vi "NPSV RTFIFO test.vi"() -> ()   [LabVIEW 2019]
uses:
  DataDef.ctl
  <vilib>/NI/Modbus Library/API/Modbus API.lvclass
  <vilib>/WPC Systems Ltd/GECO Driver/Lib/GECOBase/GECO_Driver Class/GECO_Driver.lvclass
  <vilib>/WPC Systems Ltd/GECO Driver/Lib/GECOMotion/GECOMotion/_typedefine/Axis Select.ctl
  <vilib>/WPC Systems Ltd/GECO Driver/Lib/GECOBase/GECO_Driver Class/Motion/_typedefine/GECO_Stepper Output Configuration.ctl
  <vilib>/WPC Systems Ltd/GECO Driver/Lib/GECOBase/GECO_Driver Class/Motion/_typedefine/GECO_Motion Operation Mode.ctl
  <vilib>/WPC Systems Ltd/GECO Driver/Lib/GECOBase/GECO_Driver Class/GECO_SlotName.ctl
  <vilib>/WPC Systems Ltd/GECO Driver/Lib/GECOBase/GECO_Driver Class/Motion/_typedefine/GECO_ActiveHighLow.ctl
  <vilib>/WPC Systems Ltd/GECO Driver/Lib/GECOMotion/GECOMotion/GECO Motion.lvclass
  GyroDef.ctl
  <vilib>/Platform/TimedLoop/XDataNode/timing_clust.ctl
  <vilib>/Platform/TimedLoop/XDataNode/nitl_modes.ctl
  <vilib>/Platform/TimedLoop/XDataNode/wakeup.ctl
  <vilib>/NI/Modbus Library/API/Slave/Modbus Slave.lvclass
  C:/Program Files (x86)/National Instruments/LabVIEW 2019/vi.lib/NI/Modbus Library/API/Modbus API.lvclass
  <vilib>/addons/control/pid/pid.llb/PID (DBL).vi
  <vilib>/NI/Modbus Library/API/Wrapper/Create TCP Slave.vi
  <vilib>/WPC Systems Ltd/GECO Driver/GECODriver/GECO_Initialize_RT/Initialize VIs/Initialize_GECOUnoRT_4HX.vi
  <vilib>/platform/TimedLoop/XDataNode/XDataNode.xnode
  <vilib>/addons/control/pid/NI_PID_pid.lvlib
  <vilib>/NI/Modbus Library/API/Wrapper/API Main.lvlib
  <vilib>/Platform/TimedLoop/XDataNode/XDNodeRunTimeDep.lvlib
panel:
  out "error out":errorcluster
  out "Axis 1":T1
  out "Axis 2":T1
  out "Axis 3":T1
  out "Program Period":u32
  in  "Main Setting Tab":T2(tab)
  in  "PID gains setting Tab":enum32{"Axis 1", "Axis 2", "Axis 3"}(tab)
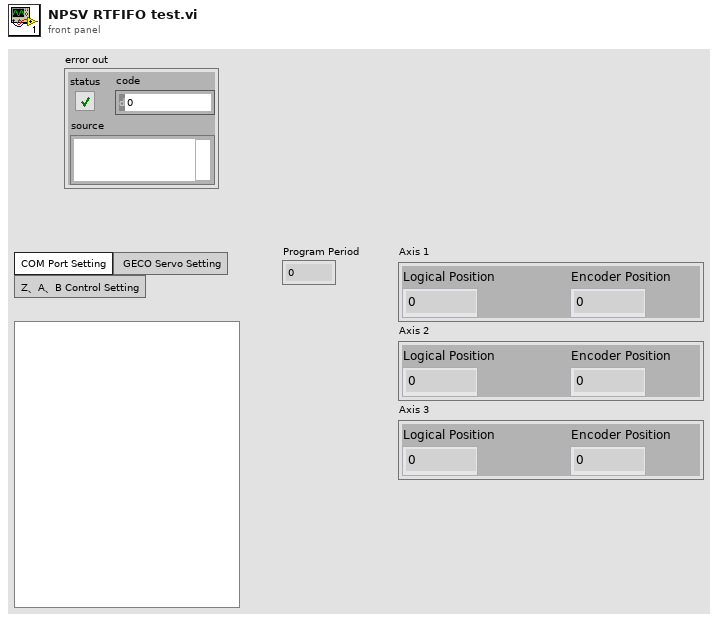
[diagram p1: front panel]
types:
  T1 = cluster{"Encoder Position":i32, "Logical Position":i32}
  T2 = enum32{"COM Port Setting", " GECO Servo Setting", "Z、A、B Control Setting"}
  T3 = typedef "DataDef.ctl" = cluster{"address starting":u16, "狀態":enum16{"初始化", "讀取", "寫入", "停止"}, "理想角度":cluster{"A":dbl, "B":dbl}, "register values":i16[], "Modbus COM":refnum<class "Modbus API.lvclass">, "TCP slave port":u16, " baud rate":u32, "Byte bits":u16, "ServoButtonControl":cluster{"三軸同退":bool, "三軸同進":bool, "三軸後退":bool, "三軸前進":bool, "二軸後退":bool, "二軸前進":bool, "一軸後退":bool, "一軸前進":bool}, "Serial Number":string, "GECO_Driver out":refnum<class "GECO_Driver.lvclass">, "number of inputs":u16, "ServoSetting":cluster{"Axis Select":T4, "Stepper Output Configuration":T5, "Motion Operation Mode":T6, "Motion Controller Slot":T7, "Singel Axis Move Paramters":cluster{"Motion Operation Mode":T6, "Target Position (0)":i32, "Velocity (10000)":i32, "Acceleration (100000)":u32, "Deacceleration (100000)":u32}, "Reverse":cluster{"Reverse Enable":bool, "Reverse Polarity":T8}, "Forward":cluster{"Forward Enable":bool, "Forward Polarity":T8}}, "GECO Motion out":refnum<class "GECO Motion.lvclass">, "Servo on":bool, "Axis 1 Position":cluster{"Encoder Position":i32, "Logical Position":i32}, "Axis 2 Position":cluster{"Encoder Position":i32, "Logical Position":i32}, "Axis 3 Position":cluster{"Encoder Position":i32, "Logical Position":i32}, "PIDSetting":cluster{"Z":i32, "A":i32, "B":i32, "Move Setting":T9, "Axis Pulse":dbl, "Axis Length":dbl, "PID gains ":cluster{"proportional gain (Kc)":dbl, "integral time (Ti, min)":dbl, "derivative time (Td, min)":dbl}}, "resource name":tag, "Save Path":refnum<file>}
  T4 = typedef "GECO Motion.lvclass/Axis Select.ctl" = enum16{"Axis 1", "Axis 2", "Axis 3", "Axis 4"}
  T5 = typedef "GECO_Driver.lvclass/GECO_Stepper Output Configuration.ctl" = enum16{"Step/Dir(One Pulse)", "CW/CCW(Two Pulse)"}
  T6 = typedef "GECO_Driver.lvclass/GECO_Motion Operation Mode.ctl" = enum16{"Absolute Position", "Relative Position", "Velocity"}
  T7 = typedef "GECO_Driver.lvclass/GECO_SlotName.ctl" = enum16{"C1", "C2", "C3", "C4"}
  T8 = typedef "GECO_Driver.lvclass/GECO_ActiveHighLow.ctl" = enum16{"Active High", "Active Low"}
  T9 = typedef "­y¸ñ.ctl" = u16
  T10 = typedef "GyroDef.ctl" = cluster{"Byte bits":u16, "baud rate":u32, "實際角度":cluster{"A":dbl, "B":dbl}, "COM Port":refnum<visa-resource-name>, "Save Path":refnum<file>}
  T11 = typedef "XDNodeRunTimeDep.lvlib/timing_clust.ctl" = cluster{"Expected End [f-1]":u64, "Actual End [f-1]":u64, "Finished Late? [f-1]":bool, "Expected End [i-1]":u64, "Actual End [i-1]":u64, "Finished Late? [i-1]":bool, "Expected Start [i]":u64, "Actual Start [i]":u64, "Expected Start [f]":u64, "Actual Start [f]":u64, "Source Name":string, "Structure Name":string, "Period":i64, "Deadline":i64, "Offset":i64, "Start":i64, "Priority":i32, "Timeout":i32, "Mode":T12, "Wakeup Reason":T13, "Error":errorcluster, "Source Type":string, "Secondary Source Type":string, "Global End Time":u64, "Global Start Time":u64, "Frame Duration":u64, "Iteration Duration":u64, "Assigned CPU":i32, "I/O Scan Engine Mode":u32}
  T12 = typedef "XDNodeRunTimeDep.lvlib/nitl_modes.ctl" = enum32{"No Change", "Process missed periods, maintain original phase", "Discard missed periods, maintain original phase", "Process missed periods, ignore original phase", "Discard missed periods, ignore original phase"}
  T13 = typedef "XDNodeRunTimeDep.lvlib/wakeup.ctl" = enum32{"Normal", "Aborted", "Asynchronous wakeup", "Timing source error", "Timed loop error", "Timeout"}
  T14 = cluster{"Motion Operation Mode":T6, "Target Position (0)":i32, "Velocity (10000)":i32, "Acceleration (100000)":u32, "Deacceleration (100000)":u32}
  T15 = cluster{"Forward Enable":bool, "Forward Polarity":T8}
  T16 = cluster{"Reverse Enable":bool, "Reverse Polarity":T8}
  T17 = cluster{"三軸同退":bool, "三軸同進":bool, "三軸後退":bool, "三軸前進":bool, "二軸後退":bool, "二軸前進":bool, "一軸後退":bool, "一軸前進":bool, "Reset Encoder Position":bool, "AlarmReset":bool}[]
  T18 = cluster{"三軸同退":bool, "三軸同進":bool, "三軸後退":bool, "三軸前進":bool, "二軸後退":bool, "二軸前進":bool, "一軸後退":bool, "一軸前進":bool, "Reset Encoder Position":bool, "AlarmReset":bool}
  T19 = enum16{"open", "replace", "create", "open or create", "replace or create", "replace or create with confirmation"}
  T20 = cluster{"Logical Position":i32, "Encoder Position":i32}
  T21 = enum16{"Step/Dir(One Pulse)", "CW/CCW(Two Pulse)"}
  T22 = enum16{"Absolute Position", "Relative Position", "Velocity"}
  T23 = cluster{"proportional gain (Kc)":dbl, "integral time (Ti, min)":dbl, "derivative time (Td, min)":dbl}
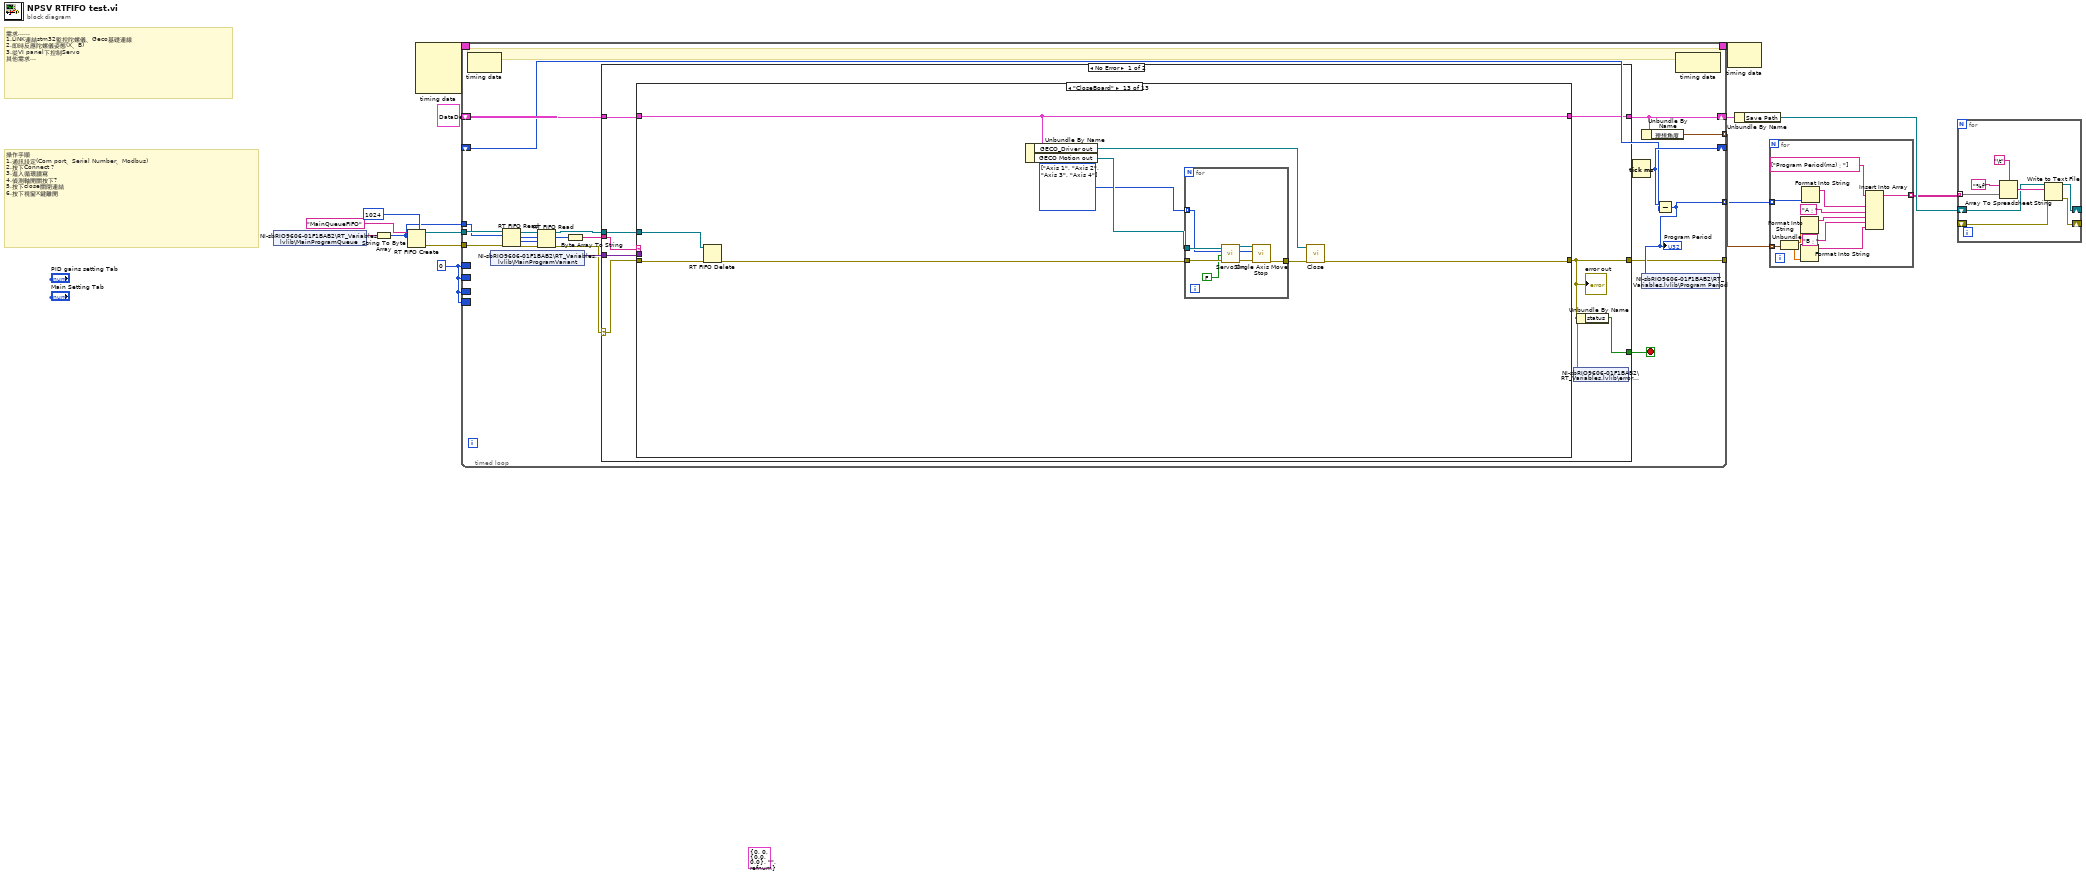
[diagram p0: block diagram]
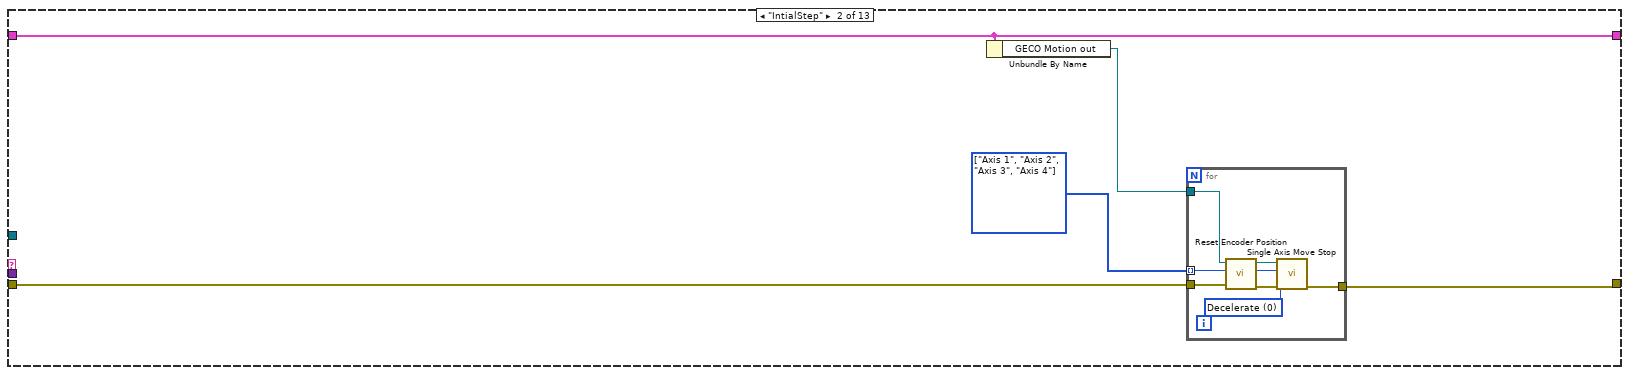
[diagram p3: hidden frame]
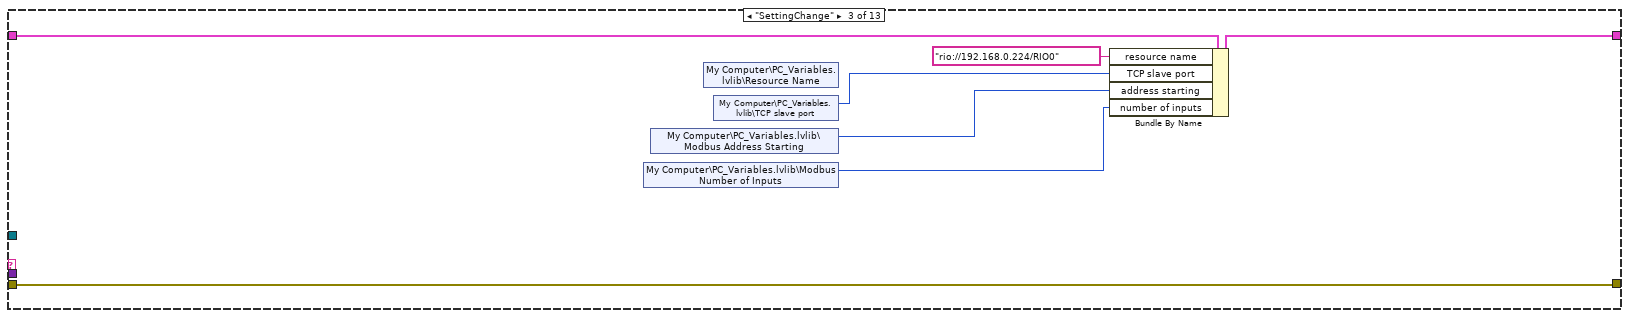
[diagram p4: hidden frame]
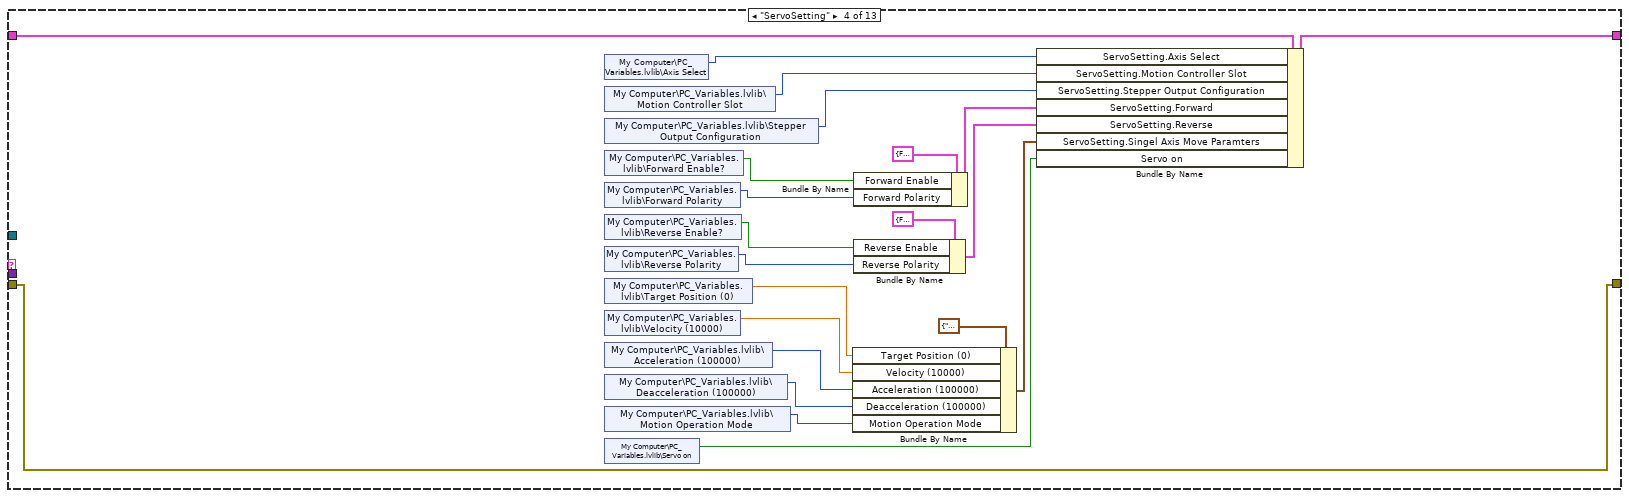
[diagram p5: hidden frame]
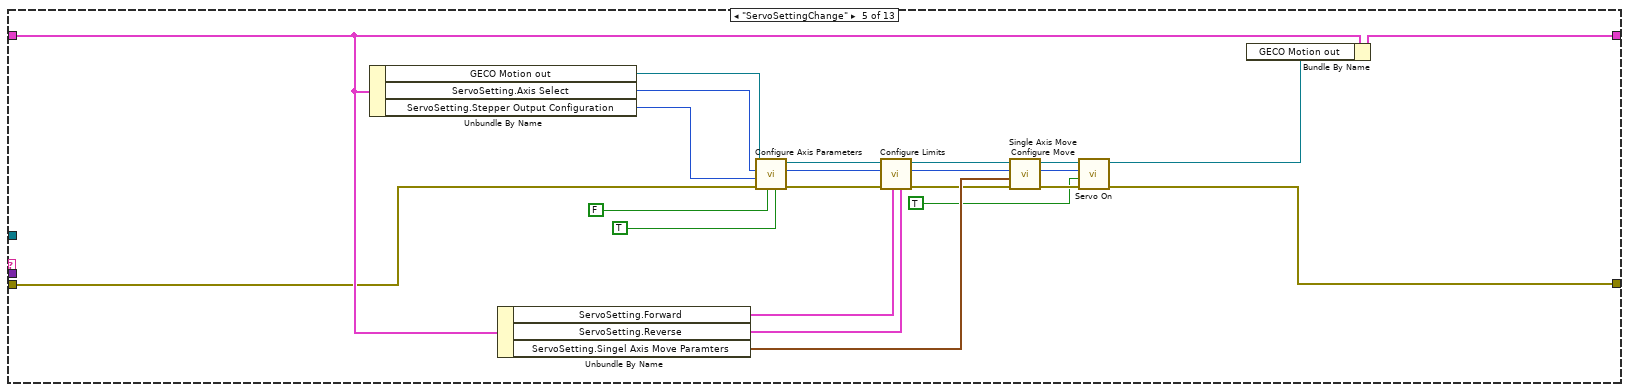
[diagram p6: hidden frame]
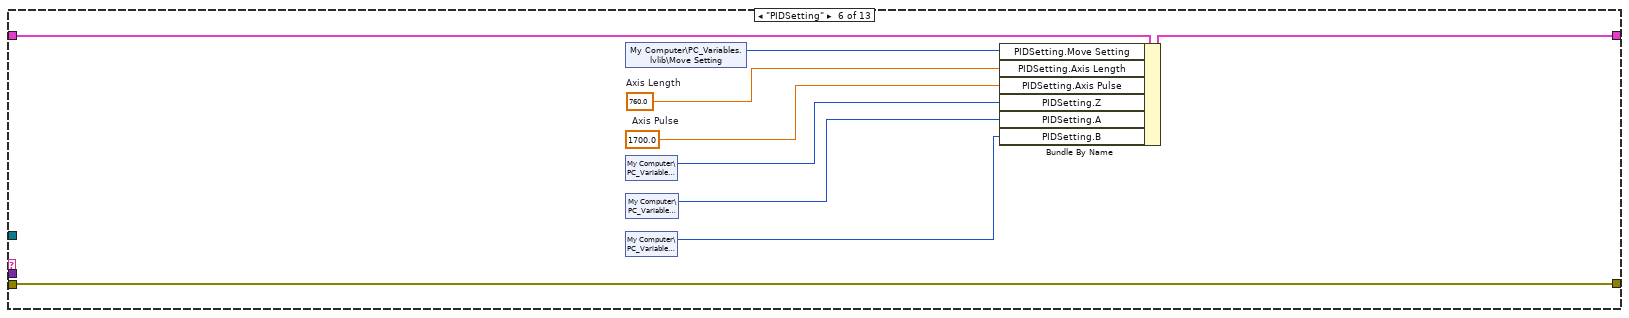
[diagram p7: hidden frame]
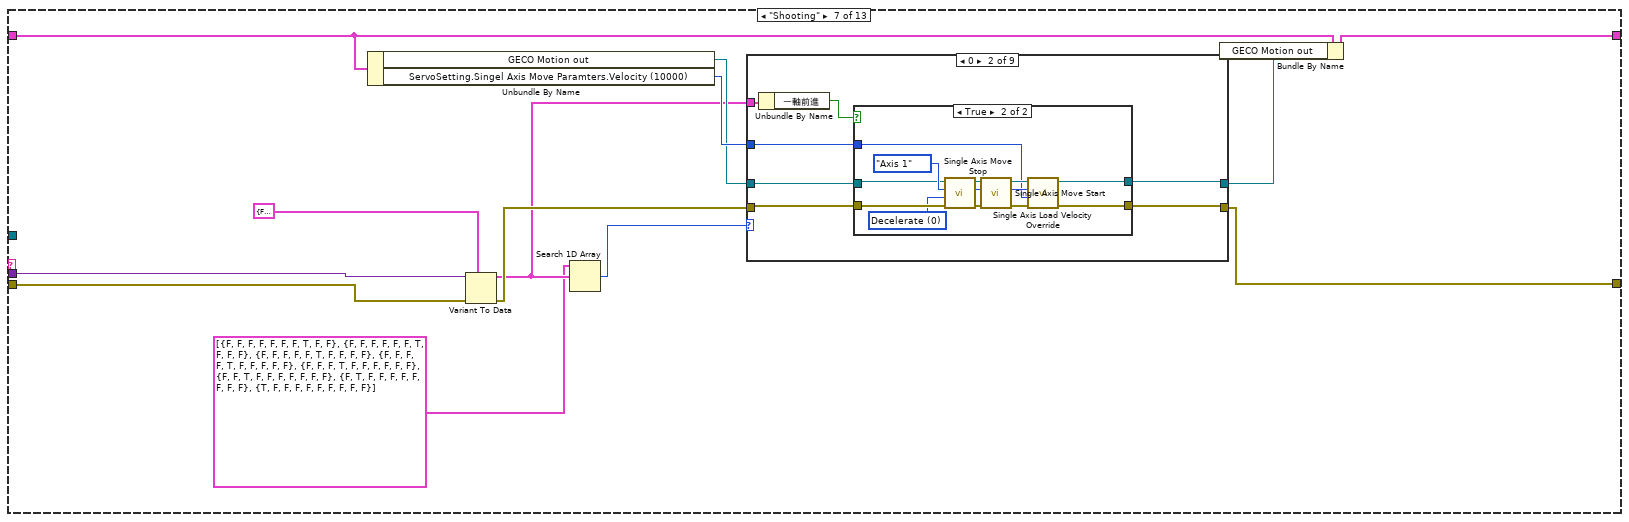
[diagram p8: hidden frame]
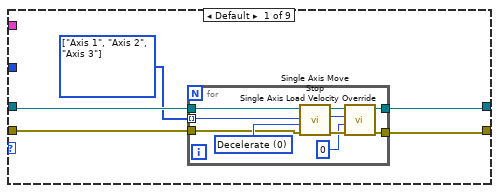
[diagram p9: hidden frame]
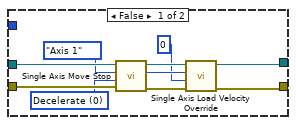
[diagram p10: hidden frame]
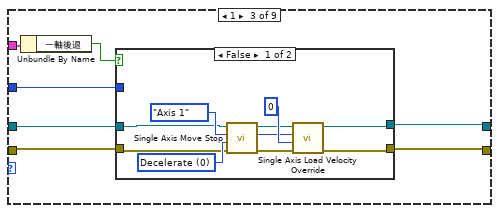
[diagram p11: hidden frame]
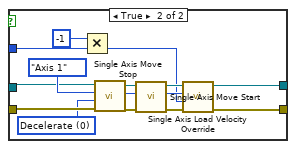
[diagram p12: hidden frame]
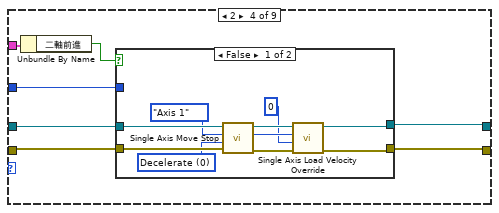
[diagram p13: hidden frame]
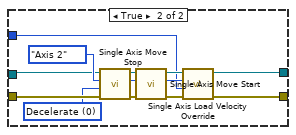
[diagram p14: hidden frame]
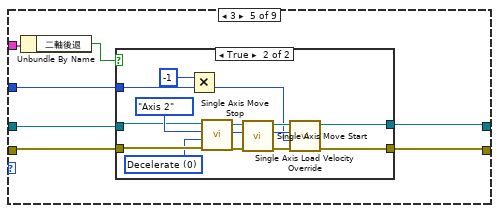
[diagram p15: hidden frame]
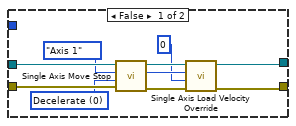
[diagram p16: hidden frame]
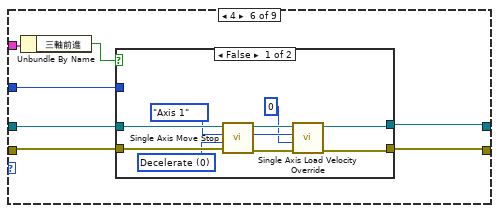
[diagram p17: hidden frame]
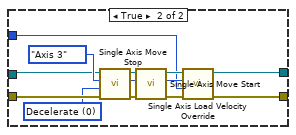
[diagram p18: hidden frame]
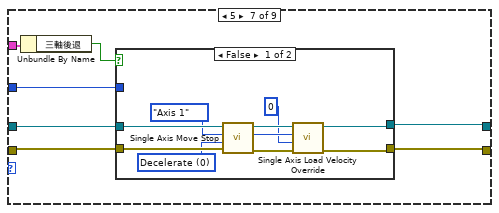
[diagram p19: hidden frame]
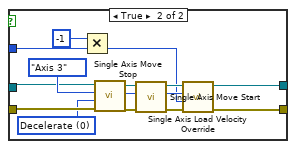
[diagram p20: hidden frame]
diagram:
  w14 = 0
  (unwired) T10 {"Byte bits"=0, "baud rate"=0, "實際角度"={"A"=0.0, "B"=0.0}, "COM Port"="", "Save Path"=refnum}
  # "操作手順\n1.通訊設定(Com port、Serial Number、Modbus)\n2.按下Connect ?\n3.進入循環讀寫\n4.偵測軸開關按下?\n5.按下close關閉連結\n6.按下視窗X鍵離開"
  # "需求......\n1.LINK連結stm32監控陀螺儀、Geco基礎連線\n2.即時反應陀螺儀姿態(X、B)\n3.從VI panel下控制Servo\n其他需求..."
  n1 = shared-variable "NI-sbRIO9606-01F1BAB2\\RT_Variables.lvlib\\MainProgramQueue"() -> (w3:string)  [unwired: 1 in, 1 out]
  n2 = String To Byte Array(string=w3) -> (unsigned byte array=w1:u8[])
  n3 = RT FIFO Create(0:"MainQueueFIFO" ("name (unnamed)"), 1:w1, 6:u32 1024 ("elements in array (1)")) -> (8:w6:refnum<k33>, 11:w2:errorcluster)  [unwired: 5 in, 1 out]
  n4 = node-c288() -> (w8:T11)  [unwired: 4 in]
  n5 = timed-loop {
    shift-right: [w31] -> w11
    shift-left: T3 {"address starting"=0, "狀態"=enum."初始化", "理想角度"={"A"=0.0, "B"=0.0}, "register values"=[], "Modbus COM"=refnum, "TCP slave port"=1, " baud rate"=0, "Byte bits"=0, "ServoButtonControl"={"三軸同退"=FALSE, "三軸同進"=FALSE, "三軸後退"=FALSE, "三軸前進"=FALSE, "二軸後退"=FALSE, "二軸前進"=FALSE, "一軸後退"=FALSE, "一軸前進"=FALSE}, "Serial Number"="", "GECO_Driver out"=refnum, "number of inputs"=0, "ServoSetting"={"Axis Select"=enum."Axis 1", "Stepper Output Configuration"=enum."Step/Dir(One Pulse)", "Motion Operation Mode"=enum."Absolute Position", "Motion Controller Slot"=enum."C1", "Singel Axis Move Paramters"={"Motion Operation Mode"=enum."Velocity", "Target Position (0)"=10000, "Velocity (10000)"=1, "Acceleration (100000)"=100000, "Deacceleration (100000)"=1}, "Reverse"={"Reverse Enable"=FALSE, "Reverse Polarity"=enum."Active Low"}, "Forward"={"Forward Enable"=FALSE, "Forward Polarity"=enum."Active Low"}}, "GECO Motion out"=refnum, "Servo on"=FALSE, "Axis 1 Position"={"Encoder Position"=0, "Logical Position"=0}, "Axis 2 Position"={"Encoder Position"=0, "Logical Position"=0}, "Axis 3 Position"={"Encoder Position"=0, "Logical Position"=0}, "PIDSetting"={"Z"=10000, "A"=10000, "B"=10000, "Move Setting"=1, "Axis Pulse"=10000.0, "Axis Length"=10000.0, "PID gains "={"proportional gain (Kc)"=1.0, "integral time (Ti, min)"=0.01, "derivative time (Td, min)"=0.0}}, "resource name"="", "Save Path"=refnum} -> [w34]
    shift-right: [w33] -> _
    shift-left: _ -> [w32]
    border: w14 -> [_]
    border: w14 -> [_]
    border: w14 -> [_]
    border: w14 -> [_]
    tunnel: [w30] -> w13 mode=indexing
    tunnel: [w29] -> w12 mode=indexing
    tunnel: [w28] -> _
    timing: w8 -> [_]
    timing-out: [_] -> w7
    tunnel: w6 -> [w18]
    tunnel: w2 -> [w19]
    tunnel: w1 -> [w17]
    stop <- w35 stop-if-true
    # "Process"
    n6 = node-c288() -> ()  [unwired: 1 in, 1 out]
    n7 = shared-variable "NI-sbRIO9606-01F1BAB2\\RT_Variables.lvlib\\MainProgramVariant"() -> (w27:variant)  [unwired: 1 in, 1 out]
    n8 = RT FIFO Read(0:w18, 1:w17, 3:w19) -> (7:w20:u32, 8:w23:refnum<k33>, 9:w21:u8[], 11:w22:errorcluster)  [unwired: 1 in, 1 out]
    n9 = RT FIFO Read(0:w23, 1:w21, 2:w20, 3:w22) -> (8:w25:refnum<k33>, 9:w16:u8[], 11:w24:errorcluster)  [unwired: 2 out]
    n10 = Byte Array To String(unsigned byte array=w16) -> (string=w26:string)
    n11 = case shown="No Error" w24 {
      selector: w24 -> [w43 w649]
      tunnel: [w42 TRUE] -> w35
      tunnel: [w45 w650] -> w31
      tunnel: w34 -> [w44 w650]
      tunnel: [w41 w649] -> w28
      tunnel: w27 -> [w40 _]
      tunnel: w26 -> [w39 _]
      tunnel: w25 -> [w38 _]
      frame No Error {
        n12 = case shown="\"CloseBoard\"" w39 {
          tunnel: [w47 w49 w66 w88 w112 w120 w132 w422 w556 w572 w605 w627 w640] -> w45
          tunnel: w44 -> [w47 w49 w67 w89 w111 w121 w126 w424 w559 w575 w606 w629 w640]
          tunnel: w43 -> [w46 w48 w63 w68 w104 w113 w134 w415 w558 w574 w588 w631 w633]
          tunnel: [w46 w52 w63 w68 w98 w113 w125 w423 w554 w570 w600 w630 w639] -> w41
          tunnel: w40 -> [_ _ _ _ _ _ w133 _ _ _ _ _ _]
          tunnel: w38 -> [_ _ _ _ _ _ _ _ _ _ _ _ w632]
          frame Default {
          }
          frame "IntialStep" {
            w50 = T4[] [enum."Axis 1", enum."Axis 2", enum."Axis 3", enum."Axis 4"] items=["Axis 1", "Axis 2", "Axis 3", "Axis 4"]
            n13 = Unbundle By Name(w49) -> ("GECO Motion out"=w51:refnum<class "GECO Motion.lvclass">)
            n14 = for {
              tunnel: [w55] -> w52
              tunnel: w51 -> [w60]
              tunnel: w50 -> [w59] mode=indexing
              tunnel: w48 -> [w53]
              w54 = u16 0 items=["Decelerate", "Halt"] ("Motion Stop Type")
              n15 = call <vilib>:"Reset Encoder Position.vi"("error in (no error)"=w53, "Axis Select"=w59, "GECO Motion in"=w60) -> ("error out"=w58:errorcluster, "Axis Select out"=w57:T4, "GECO Motion out"=w56:refnum<class "GECO Motion.lvclass">)  [unwired: 6 in]
              n16 = call <vilib>:"Single Axis Move Stop.vi"("error in (no error)"=w58, "Motion Stop Type"=w54, "Axis Select"=w57, "GECO Motion in"=w56) -> ("error out"=w55:errorcluster)  [unwired: 5 in, 2 out]
            }
          }
          frame "SettingChange" {
            n17 = shared-variable "My Computer\\PC_Variables.lvlib\\Modbus Number of Inputs"() -> (w62:u32)  [unwired: 1 in, 1 out]
            n18 = shared-variable "My Computer\\PC_Variables.lvlib\\Modbus Address Starting"() -> (w64:u32)  [unwired: 1 in, 1 out]
            n19 = shared-variable "My Computer\\PC_Variables.lvlib\\Resource Name"() -> ()  [unwired: 1 in, 2 out]
            n20 = shared-variable "My Computer\\PC_Variables.lvlib\\TCP slave port"() -> (w65:u32)  [unwired: 1 in, 1 out]
            n21 = Bundle By Name(cluster=w67, "resource name"=tag "rio://192.168.0.224/RIO0", "TCP slave port"=w65, "address starting"=w64, "number of inputs"=w62) -> (w66:T3)
          }
          frame "ServoSetting" {
            n22 = shared-variable "My Computer\\PC_Variables.lvlib\\Axis Select"() -> (w87:enum16{"Axis 1", "Axis 2", "Axis 3", "Axis 4"})  [unwired: 1 in, 1 out]
            n23 = shared-variable "My Computer\\PC_Variables.lvlib\\Motion Controller Slot"() -> (w86:enum16{"C1", "C2", "C3", "C4"})  [unwired: 1 in, 1 out]
            n24 = shared-variable "My Computer\\PC_Variables.lvlib\\Stepper Output Configuration"() -> (w85:T21)  [unwired: 1 in, 1 out]
            n25 = shared-variable "My Computer\\PC_Variables.lvlib\\Forward Enable?"() -> (w73:bool)  [unwired: 1 in, 1 out]
            n26 = shared-variable "My Computer\\PC_Variables.lvlib\\Forward Polarity"() -> (w74:enum16{"Active High", "Active Low"})  [unwired: 1 in, 1 out]
            n27 = shared-variable "My Computer\\PC_Variables.lvlib\\Reverse Enable?"() -> (w76:bool)  [unwired: 1 in, 1 out]
            n28 = shared-variable "My Computer\\PC_Variables.lvlib\\Reverse Polarity"() -> (w75:enum16{"Active High", "Active Low"})  [unwired: 1 in, 1 out]
            n29 = shared-variable "My Computer\\PC_Variables.lvlib\\Target Position (0)"() -> (w77:dbl)  [unwired: 1 in, 1 out]
            n30 = shared-variable "My Computer\\PC_Variables.lvlib\\Velocity (10000)"() -> (w78:dbl)  [unwired: 1 in, 1 out]
            n31 = shared-variable "My Computer\\PC_Variables.lvlib\\Acceleration (100000)"() -> (w79:u32)  [unwired: 1 in, 1 out]
            n32 = shared-variable "My Computer\\PC_Variables.lvlib\\Deacceleration (100000)"() -> (w80:u32)  [unwired: 1 in, 1 out]
            n33 = shared-variable "My Computer\\PC_Variables.lvlib\\Motion Operation Mode"() -> (w81:T22)  [unwired: 1 in, 1 out]
            n34 = shared-variable "My Computer\\PC_Variables.lvlib\\Servo on"() -> (w69:bool)  [unwired: 1 in, 1 out]
            n35 = Bundle By Name(cluster=T14 {"Motion Operation Mode"=enum."Absolute Position", "Target Position (0)"=0, "Velocity (10000)"=10000, "Acceleration (100000)"=100000, "Deacceleration (100000)"=100000} ("Singel Axis Move Paramters"), "Target Position (0)"=w77, "Velocity (10000)"=w78, "Acceleration (100000)"=w79, "Deacceleration (100000)"=w80, "Motion Operation Mode"=w81) -> (w70:T14)
            n36 = Bundle By Name(cluster=T15 {"Forward Enable"=FALSE, "Forward Polarity"=enum."Active Low"} ("Forward"), "Forward Enable"=w73, "Forward Polarity"=w74) -> (w72:T15)
            n37 = Bundle By Name(cluster=T16 {"Reverse Enable"=FALSE, "Reverse Polarity"=enum."Active Low"} ("Reverse"), "Reverse Enable"=w76, "Reverse Polarity"=w75) -> (w71:T16)
            n38 = Bundle By Name(cluster=w89, "ServoSetting.Axis Select"=w87, "ServoSetting.Motion Controller Slot"=w86, "ServoSetting.Stepper Output Configuration"=w85, "ServoSetting.Forward"=w72, "ServoSetting.Reverse"=w71, "ServoSetting.Singel Axis Move Paramters"=w70, "Servo on"=w69) -> (w88:T3)
          }
          frame "ServoSettingChange" {
            n39 = Unbundle By Name(w111) -> ("GECO Motion out"=w105:refnum<class "GECO Motion.lvclass">, "ServoSetting.Axis Select"=w109:T4, "ServoSetting.Stepper Output Configuration"=w108:T5)
            n40 = Unbundle By Name(w111) -> ("ServoSetting.Forward"=w91:T15, "ServoSetting.Reverse"=w90:T16, "ServoSetting.Singel Axis Move Paramters"=w110:T14)
            n41 = call <vilib>:"Configure Axis Parameters.vi"("Reverse Encoder Direction?"=TRUE, "Reverse Axis Direction?"=FALSE, "error in (no error)"=w104, "Stepper Output Configuration"=w108, "Axis Select"=w109, "GECO Motion in"=w105) -> ("error out"=w95:errorcluster, "Axis Select out"=w97:T4, "GECO Motion out"=w96:refnum<class "GECO Motion.lvclass">)  [unwired: 3 in]
            n42 = call <vilib>:"Configure Limits.vi"("Reverse"=w90, "Forward"=w91, "error in (no error)"=w95, "Axis Select"=w97, "GECO Motion in"=w96) -> ("error out"=w92:errorcluster, "Axis Select out"=w93:T4, "GECO Motion out"=w94:refnum<class "GECO Motion.lvclass">)  [unwired: 4 in]
            n43 = call <vilib>:"Single Axis Move Configure Move.vi"("error in (no error)"=w92, "Singel Axis Move Paramters"=w110, "Axis Select"=w93, "GECO Motion in"=w94) -> ("error out"=w101:errorcluster, "Axis Select out"=w102:T4, "GECO Motion out"=w103:refnum<class "GECO Motion.lvclass">)  [unwired: 5 in]
            n44 = call <vilib>:"Servo On.vi"("error in (no error)"=w101, "Servo On"=TRUE, "Axis Select"=w102, "GECO Motion in"=w103) -> ("error out"=w98:errorcluster, "GECO Motion out"=w99:refnum<class "GECO Motion.lvclass">)  [unwired: 5 in, 1 out]
            n45 = Bundle By Name(cluster=w111, "GECO Motion out"=w99) -> (w112:T3)
          }
          frame "PIDSetting" {
            w117 = 1700.0  # Axis Pulse
            w118 = 760.0  # Axis Length
            n46 = shared-variable "My Computer\\PC_Variables.lvlib\\Move Setting"() -> (w119:u16)  [unwired: 1 in, 1 out]
            n47 = shared-variable "My Computer\\PC_Variables.lvlib\\Z"() -> (w116:i32)  [unwired: 1 in, 1 out]
            n48 = shared-variable "My Computer\\PC_Variables.lvlib\\A"() -> (w115:i32)  [unwired: 1 in, 1 out]
            n49 = shared-variable "My Computer\\PC_Variables.lvlib\\B"() -> (w114:i32)  [unwired: 1 in, 1 out]
            n50 = Bundle By Name(cluster=w121, "PIDSetting.Move Setting"=w119, "PIDSetting.Axis Length"=w118, "PIDSetting.Axis Pulse"=w117, "PIDSetting.Z"=w116, "PIDSetting.A"=w115, "PIDSetting.B"=w114) -> (w120:T3)
          }
          frame "Shooting" {
            n51 = Unbundle By Name(w126) -> ("GECO Motion out"=w128:refnum<class "GECO Motion.lvclass">, "ServoSetting.Singel Axis Move Paramters.Velocity (10000)"=w129:i32)
            n52 = Variant To Data(error in=w134, type=T18 {"三軸同退"=FALSE, "三軸同進"=FALSE, "三軸後退"=FALSE, "三軸前進"=FALSE, "二軸後退"=FALSE, "二軸前進"=FALSE, "一軸後退"=FALSE, "一軸前進"=FALSE, "Reset Encoder Position"=FALSE, "AlarmReset"=FALSE} ("ServoButtonControl"), Variant=w133) -> (data=w124:T18, error out=w130:errorcluster)
            n53 = Search 1D Array(1D array=T17 [{"三軸同退"=FALSE, "三軸同進"=FALSE, "三軸後退"=FALSE, "三軸前進"=FALSE, "二軸後退"=FALSE, "二軸前進"=FALSE, "一軸後退"=FALSE, "一軸前進"=TRUE, "Reset Encoder Position"=FALSE, "AlarmReset"=FALSE}, {"三軸同退"=FALSE, "三軸同進"=FALSE, "三軸後退"=FALSE, "三軸前進"=FALSE, "二軸後退"=FALSE, "二軸前進"=FALSE, "一軸後退"=TRUE, "一軸前進"=FALSE, "Reset Encoder Position"=FALSE, "AlarmReset"=FALSE}, {"三軸同退"=FALSE, "三軸同進"=FALSE, "三軸後退"=FALSE, "三軸前進"=FALSE, "二軸後退"=FALSE, "二軸前進"=TRUE, "一軸後退"=FALSE, "一軸前進"=FALSE, "Reset Encoder Position"=FALSE, "AlarmReset"=FALSE}, {"三軸同退"=FALSE, "三軸同進"=FALSE, "三軸後退"=FALSE, "三軸前進"=FALSE, "二軸後退"=TRUE, "二軸前進"=FALSE, "一軸後退"=FALSE, "一軸前進"=FALSE, "Reset Encoder Position"=FALSE, "AlarmReset"=FALSE}, {"三軸同退"=FALSE, "三軸同進"=FALSE, "三軸後退"=FALSE, "三軸前進"=TRUE, "二軸後退"=FALSE, "二軸前進"=FALSE, "一軸後退"=FALSE, "一軸前進"=FALSE, "Reset Encoder Position"=FALSE, "AlarmReset"=FALSE}, {"三軸同退"=FALSE, "三軸同進"=FALSE, "三軸後退"=TRUE, "三軸前進"=FALSE, "二軸後退"=FALSE, "二軸前進"=FALSE, "一軸後退"=FALSE, "一軸前進"=FALSE, "Reset Encoder Position"=FALSE, "AlarmReset"=FALSE}, {"三軸同退"=FALSE, "三軸同進"=TRUE, "三軸後退"=FALSE, "三軸前進"=FALSE, "二軸後退"=FALSE, "二軸前進"=FALSE, "一軸後退"=FALSE, "一軸前進"=FALSE, "Reset Encoder Position"=FALSE, "AlarmReset"=FALSE}, {"三軸同退"=TRUE, "三軸同進"=FALSE, "三軸後退"=FALSE, "三軸前進"=FALSE, "二軸後退"=FALSE, "二軸前進"=FALSE, "一軸後退"=FALSE, "一軸前進"=FALSE, "Reset Encoder Position"=FALSE, "AlarmReset"=FALSE}], element=w124) -> (index of element=w131:i32)  [unwired: 1 in]
            n54 = case shown="0" w131 {
              tunnel: w130 -> [w138 w155 w185 w217 w247 w279 w309 w341 w378]
              tunnel: w129 -> [_ w154 w184 w216 w246 w278 w308 w340 w377]
              tunnel: w128 -> [w139 w156 w186 w218 w248 w280 w310 w342 w379]
              tunnel: [w136 w153 w183 w215 w245 w277 w307 w339 w376] -> w127
              tunnel: [w135 w152 w182 w214 w244 w276 w306 w338 w375] -> w125
              tunnel: w124 -> [_ w151 w181 w213 w243 w275 w305 w337 w374]
              frame Default {
                w137 = T4[] [enum."Axis 1", enum."Axis 2", enum."Axis 3"] items=["Axis 1", "Axis 2", "Axis 3", "Axis 4"] ("Start Axes Select")
                n55 = for {
                  tunnel: w138 -> [w148]
                  tunnel: w139 -> [w147]
                  tunnel: w137 -> [w146] mode=indexing
                  tunnel: [w141] -> w136
                  tunnel: [w142] -> w135
                  w149 = u16 0 items=["Decelerate", "Halt"] ("Motion Stop Type")
                  n56 = call <vilib>:"Single Axis Move Stop.vi"("error in (no error)"=w148, "Motion Stop Type"=w149, "Axis Select"=w146, "GECO Motion in"=w147) -> ("error out"=w144:errorcluster, "Axis Select out"=w143:T4, "GECO Motion out"=w145:refnum<class "GECO Motion.lvclass">)  [unwired: 5 in]
                  n57 = call <vilib>:"Single Axis Load Velocity Override.vi"("error in (no error)"=w144, "Override Velosity Value"=0, "Axis Select"=w143, "GECO Motion in"=w145) -> ("error out"=w142:errorcluster, "GECO Motion out"=w141:refnum<class "GECO Motion.lvclass">)  [unwired: 5 in, 1 out]
                }
              }
              frame 0 {
                n58 = Unbundle By Name(w151) -> ("一軸前進"=w150:bool)
                n59 = case shown="True" w150 {
                  tunnel: w156 -> [w166 w172]
                  tunnel: w155 -> [w165 w171]
                  tunnel: w154 -> [_ w176]
                  tunnel: [w157 w175] -> w153
                  tunnel: [w158 w174] -> w152
                  frame False {
                    w164 = u16 0 items=["Decelerate", "Halt"] ("Motion Stop Type")
                    n60 = call <vilib>:"Single Axis Move Stop.vi"("error in (no error)"=w165, "Motion Stop Type"=w164, "Axis Select"=Axis_Select."Axis 1", "GECO Motion in"=w166) -> ("error out"=w161:errorcluster, "Axis Select out"=w160:T4, "GECO Motion out"=w162:refnum<class "GECO Motion.lvclass">)  [unwired: 5 in]
                    n61 = call <vilib>:"Single Axis Load Velocity Override.vi"("error in (no error)"=w161, "Override Velosity Value"=0, "Axis Select"=w160, "GECO Motion in"=w162) -> ("error out"=w158:errorcluster, "GECO Motion out"=w157:refnum<class "GECO Motion.lvclass">)  [unwired: 5 in, 1 out]
                  }
                  frame True {
                    w170 = u16 0 items=["Decelerate", "Halt"] ("Motion Stop Type")
                    n62 = call <vilib>:"Single Axis Move Stop.vi"("error in (no error)"=w171, "Motion Stop Type"=w170, "Axis Select"=Axis_Select."Axis 1", "GECO Motion in"=w172) -> ("error out"=w168:errorcluster, "Axis Select out"=w167:T4, "GECO Motion out"=w169:refnum<class "GECO Motion.lvclass">)  [unwired: 5 in]
                    n63 = call <vilib>:"Single Axis Move Start.vi"("error in (no error)"=w168, "Axis Select"=w167, "GECO Motion in"=w169) -> ("error out"=w178:errorcluster, "Axis Select out"=w177:T4, "GECO Motion out"=w179:refnum<class "GECO Motion.lvclass">)  [unwired: 6 in]
                    n64 = call <vilib>:"Single Axis Load Velocity Override.vi"("error in (no error)"=w178, "Override Velosity Value"=w176, "Axis Select"=w177, "GECO Motion in"=w179) -> ("error out"=w174:errorcluster, "GECO Motion out"=w175:refnum<class "GECO Motion.lvclass">)  [unwired: 5 in, 1 out]
                  }
                }
              }
              frame 1 {
                n65 = Unbundle By Name(w181) -> ("一軸後退"=w180:bool)
                n66 = case shown="False" w180 {
                  tunnel: w186 -> [w192 w200]
                  tunnel: w185 -> [w190 w199]
                  tunnel: w184 -> [_ w208]
                  tunnel: [w194 w207] -> w183
                  tunnel: [w195 w206] -> w182
                  frame False {
                    w191 = u16 0 items=["Decelerate", "Halt"] ("Motion Stop Type")
                    n67 = call <vilib>:"Single Axis Move Stop.vi"("error in (no error)"=w190, "Motion Stop Type"=w191, "Axis Select"=Axis_Select."Axis 1", "GECO Motion in"=w192) -> ("error out"=w188:errorcluster, "Axis Select out"=w187:T4, "GECO Motion out"=w189:refnum<class "GECO Motion.lvclass">)  [unwired: 5 in]
                    n68 = call <vilib>:"Single Axis Load Velocity Override.vi"("error in (no error)"=w188, "Override Velosity Value"=0, "Axis Select"=w187, "GECO Motion in"=w189) -> ("error out"=w195:errorcluster, "GECO Motion out"=w194:refnum<class "GECO Motion.lvclass">)  [unwired: 5 in, 1 out]
                  }
                  frame True {
                    w198 = u16 0 items=["Decelerate", "Halt"] ("Motion Stop Type")
                    n69 = Multiply(x=-1, y=w208) -> (x*y=w205:i32)
                    n70 = call <vilib>:"Single Axis Move Stop.vi"("error in (no error)"=w199, "Motion Stop Type"=w198, "Axis Select"=Axis_Select."Axis 1", "GECO Motion in"=w200) -> ("error out"=w202:errorcluster, "Axis Select out"=w197:T4, "GECO Motion out"=w203:refnum<class "GECO Motion.lvclass">)  [unwired: 5 in]
                    n71 = call <vilib>:"Single Axis Move Start.vi"("error in (no error)"=w202, "Axis Select"=w197, "GECO Motion in"=w203) -> ("error out"=w210:errorcluster, "Axis Select out"=w209:T4, "GECO Motion out"=w211:refnum<class "GECO Motion.lvclass">)  [unwired: 6 in]
                    n72 = call <vilib>:"Single Axis Load Velocity Override.vi"("error in (no error)"=w210, "Override Velosity Value"=w205, "Axis Select"=w209, "GECO Motion in"=w211) -> ("error out"=w206:errorcluster, "GECO Motion out"=w207:refnum<class "GECO Motion.lvclass">)  [unwired: 5 in, 1 out]
                  }
                }
              }
              frame 2 {
                n73 = Unbundle By Name(w213) -> ("二軸前進"=w212:bool)
                n74 = case shown="False" w212 {
                  tunnel: w218 -> [w228 w234]
                  tunnel: w217 -> [w227 w233]
                  tunnel: w216 -> [_ w238]
                  tunnel: [w219 w237] -> w215
                  tunnel: [w220 w236] -> w214
                  frame False {
                    w226 = u16 0 items=["Decelerate", "Halt"] ("Motion Stop Type")
                    n75 = call <vilib>:"Single Axis Move Stop.vi"("error in (no error)"=w227, "Motion Stop Type"=w226, "Axis Select"=Axis_Select."Axis 1", "GECO Motion in"=w228) -> ("error out"=w223:errorcluster, "Axis Select out"=w222:T4, "GECO Motion out"=w224:refnum<class "GECO Motion.lvclass">)  [unwired: 5 in]
                    n76 = call <vilib>:"Single Axis Load Velocity Override.vi"("error in (no error)"=w223, "Override Velosity Value"=0, "Axis Select"=w222, "GECO Motion in"=w224) -> ("error out"=w220:errorcluster, "GECO Motion out"=w219:refnum<class "GECO Motion.lvclass">)  [unwired: 5 in, 1 out]
                  }
                  frame True {
                    w232 = u16 0 items=["Decelerate", "Halt"] ("Motion Stop Type")
                    n77 = call <vilib>:"Single Axis Move Stop.vi"("error in (no error)"=w233, "Motion Stop Type"=w232, "Axis Select"=Axis_Select."Axis 2", "GECO Motion in"=w234) -> ("error out"=w230:errorcluster, "Axis Select out"=w229:T4, "GECO Motion out"=w231:refnum<class "GECO Motion.lvclass">)  [unwired: 5 in]
                    n78 = call <vilib>:"Single Axis Move Start.vi"("error in (no error)"=w230, "Axis Select"=w229, "GECO Motion in"=w231) -> ("error out"=w240:errorcluster, "Axis Select out"=w239:T4, "GECO Motion out"=w241:refnum<class "GECO Motion.lvclass">)  [unwired: 6 in]
                    n79 = call <vilib>:"Single Axis Load Velocity Override.vi"("error in (no error)"=w240, "Override Velosity Value"=w238, "Axis Select"=w239, "GECO Motion in"=w241) -> ("error out"=w236:errorcluster, "GECO Motion out"=w237:refnum<class "GECO Motion.lvclass">)  [unwired: 5 in, 1 out]
                  }
                }
              }
              frame 3 {
                n80 = Unbundle By Name(w243) -> ("二軸後退"=w242:bool)
                n81 = case shown="True" w242 {
                  tunnel: w248 -> [w258 w262]
                  tunnel: w247 -> [w257 w261]
                  tunnel: w246 -> [_ w270]
                  tunnel: [w249 w269] -> w245
                  tunnel: [w250 w268] -> w244
                  frame False {
                    w256 = u16 0 items=["Decelerate", "Halt"] ("Motion Stop Type")
                    n82 = call <vilib>:"Single Axis Move Stop.vi"("error in (no error)"=w257, "Motion Stop Type"=w256, "Axis Select"=Axis_Select."Axis 1", "GECO Motion in"=w258) -> ("error out"=w253:errorcluster, "Axis Select out"=w252:T4, "GECO Motion out"=w254:refnum<class "GECO Motion.lvclass">)  [unwired: 5 in]
                    n83 = call <vilib>:"Single Axis Load Velocity Override.vi"("error in (no error)"=w253, "Override Velosity Value"=0, "Axis Select"=w252, "GECO Motion in"=w254) -> ("error out"=w250:errorcluster, "GECO Motion out"=w249:refnum<class "GECO Motion.lvclass">)  [unwired: 5 in, 1 out]
                  }
                  frame True {
                    w260 = u16 0 items=["Decelerate", "Halt"] ("Motion Stop Type")
                    n84 = Multiply(x=-1, y=w270) -> (x*y=w267:i32)
                    n85 = call <vilib>:"Single Axis Move Stop.vi"("error in (no error)"=w261, "Motion Stop Type"=w260, "Axis Select"=Axis_Select."Axis 2", "GECO Motion in"=w262) -> ("error out"=w264:errorcluster, "Axis Select out"=w259:T4, "GECO Motion out"=w265:refnum<class "GECO Motion.lvclass">)  [unwired: 5 in]
                    n86 = call <vilib>:"Single Axis Move Start.vi"("error in (no error)"=w264, "Axis Select"=w259, "GECO Motion in"=w265) -> ("error out"=w272:errorcluster, "Axis Select out"=w271:T4, "GECO Motion out"=w273:refnum<class "GECO Motion.lvclass">)  [unwired: 6 in]
                    n87 = call <vilib>:"Single Axis Load Velocity Override.vi"("error in (no error)"=w272, "Override Velosity Value"=w267, "Axis Select"=w271, "GECO Motion in"=w273) -> ("error out"=w268:errorcluster, "GECO Motion out"=w269:refnum<class "GECO Motion.lvclass">)  [unwired: 5 in, 1 out]
                  }
                }
              }
              frame 4 {
                n88 = Unbundle By Name(w275) -> ("三軸前進"=w274:bool)
                n89 = case shown="False" w274 {
                  tunnel: w280 -> [w290 w296]
                  tunnel: w279 -> [w289 w295]
                  tunnel: w278 -> [_ w300]
                  tunnel: [w281 w299] -> w277
                  tunnel: [w282 w298] -> w276
                  frame False {
                    w288 = u16 0 items=["Decelerate", "Halt"] ("Motion Stop Type")
                    n90 = call <vilib>:"Single Axis Move Stop.vi"("error in (no error)"=w289, "Motion Stop Type"=w288, "Axis Select"=Axis_Select."Axis 1", "GECO Motion in"=w290) -> ("error out"=w285:errorcluster, "Axis Select out"=w284:T4, "GECO Motion out"=w286:refnum<class "GECO Motion.lvclass">)  [unwired: 5 in]
                    n91 = call <vilib>:"Single Axis Load Velocity Override.vi"("error in (no error)"=w285, "Override Velosity Value"=0, "Axis Select"=w284, "GECO Motion in"=w286) -> ("error out"=w282:errorcluster, "GECO Motion out"=w281:refnum<class "GECO Motion.lvclass">)  [unwired: 5 in, 1 out]
                  }
                  frame True {
                    w294 = u16 0 items=["Decelerate", "Halt"] ("Motion Stop Type")
                    n92 = call <vilib>:"Single Axis Move Stop.vi"("error in (no error)"=w295, "Motion Stop Type"=w294, "Axis Select"=Axis_Select."Axis 3", "GECO Motion in"=w296) -> ("error out"=w292:errorcluster, "Axis Select out"=w291:T4, "GECO Motion out"=w293:refnum<class "GECO Motion.lvclass">)  [unwired: 5 in]
                    n93 = call <vilib>:"Single Axis Move Start.vi"("error in (no error)"=w292, "Axis Select"=w291, "GECO Motion in"=w293) -> ("error out"=w302:errorcluster, "Axis Select out"=w301:T4, "GECO Motion out"=w303:refnum<class "GECO Motion.lvclass">)  [unwired: 6 in]
                    n94 = call <vilib>:"Single Axis Load Velocity Override.vi"("error in (no error)"=w302, "Override Velosity Value"=w300, "Axis Select"=w301, "GECO Motion in"=w303) -> ("error out"=w298:errorcluster, "GECO Motion out"=w299:refnum<class "GECO Motion.lvclass">)  [unwired: 5 in, 1 out]
                  }
                }
              }
              frame 5 {
                n95 = Unbundle By Name(w305) -> ("三軸後退"=w304:bool)
                n96 = case shown="False" w304 {
                  tunnel: w310 -> [w320 w324]
                  tunnel: w309 -> [w319 w323]
                  tunnel: w308 -> [_ w332]
                  tunnel: [w311 w331] -> w307
                  tunnel: [w312 w330] -> w306
                  frame False {
                    w318 = u16 0 items=["Decelerate", "Halt"] ("Motion Stop Type")
                    n97 = call <vilib>:"Single Axis Move Stop.vi"("error in (no error)"=w319, "Motion Stop Type"=w318, "Axis Select"=Axis_Select."Axis 1", "GECO Motion in"=w320) -> ("error out"=w315:errorcluster, "Axis Select out"=w314:T4, "GECO Motion out"=w316:refnum<class "GECO Motion.lvclass">)  [unwired: 5 in]
                    n98 = call <vilib>:"Single Axis Load Velocity Override.vi"("error in (no error)"=w315, "Override Velosity Value"=0, "Axis Select"=w314, "GECO Motion in"=w316) -> ("error out"=w312:errorcluster, "GECO Motion out"=w311:refnum<class "GECO Motion.lvclass">)  [unwired: 5 in, 1 out]
                  }
                  frame True {
                    w322 = u16 0 items=["Decelerate", "Halt"] ("Motion Stop Type")
                    n99 = Multiply(x=-1, y=w332) -> (x*y=w329:i32)
                    n100 = call <vilib>:"Single Axis Move Stop.vi"("error in (no error)"=w323, "Motion Stop Type"=w322, "Axis Select"=Axis_Select."Axis 3", "GECO Motion in"=w324) -> ("error out"=w326:errorcluster, "Axis Select out"=w321:T4, "GECO Motion out"=w327:refnum<class "GECO Motion.lvclass">)  [unwired: 5 in]
                    n101 = call <vilib>:"Single Axis Move Start.vi"("error in (no error)"=w326, "Axis Select"=w321, "GECO Motion in"=w327) -> ("error out"=w334:errorcluster, "Axis Select out"=w333:T4, "GECO Motion out"=w335:refnum<class "GECO Motion.lvclass">)  [unwired: 6 in]
                    n102 = call <vilib>:"Single Axis Load Velocity Override.vi"("error in (no error)"=w334, "Override Velosity Value"=w329, "Axis Select"=w333, "GECO Motion in"=w335) -> ("error out"=w330:errorcluster, "GECO Motion out"=w331:refnum<class "GECO Motion.lvclass">)  [unwired: 5 in, 1 out]
                  }
                }
              }
              frame 6 {
                n103 = Unbundle By Name(w337) -> ("三軸同進"=w336:bool)
                n104 = case shown="False" w336 {
                  tunnel: w342 -> [w346 w364]
                  tunnel: w341 -> [w347 w363]
                  tunnel: w340 -> [_ w359]
                  tunnel: [w344 w372] -> w339
                  tunnel: [w343 w371] -> w338
                  frame False {
                    w345 = T4[] [enum."Axis 1", enum."Axis 2", enum."Axis 3"] items=["Axis 1", "Axis 2", "Axis 3", "Axis 4"] ("Start Axes Select")
                    n105 = for {
                      tunnel: w347 -> [w356]
                      tunnel: w346 -> [w355]
                      tunnel: w345 -> [w354] mode=indexing
                      tunnel: [w349] -> w344
                      tunnel: [w350] -> w343
                      w357 = u16 0 items=["Decelerate", "Halt"] ("Motion Stop Type")
                      n106 = call <vilib>:"Single Axis Move Stop.vi"("error in (no error)"=w356, "Motion Stop Type"=w357, "Axis Select"=w354, "GECO Motion in"=w355) -> ("error out"=w352:errorcluster, "Axis Select out"=w351:T4, "GECO Motion out"=w353:refnum<class "GECO Motion.lvclass">)  [unwired: 5 in]
                      n107 = call <vilib>:"Single Axis Load Velocity Override.vi"("error in (no error)"=w352, "Override Velosity Value"=0, "Axis Select"=w351, "GECO Motion in"=w353) -> ("error out"=w350:errorcluster, "GECO Motion out"=w349:refnum<class "GECO Motion.lvclass">)  [unwired: 5 in, 1 out]
                    }
                  }
                  frame True {
                    w360 = T4[] [enum."Axis 1", enum."Axis 2", enum."Axis 3"] items=["Axis 1", "Axis 2", "Axis 3", "Axis 4"] ("Start Axes Select")
                    n108 = call <vilib>:"Single Axis Load Velocity Override.vi"("error in (no error)"=w363, "Override Velosity Value"=w359, "Axis Select"=Axis_Select."Axis 1", "GECO Motion in"=w364) -> ("error out"=w369:errorcluster, "GECO Motion out"=w370:refnum<class "GECO Motion.lvclass">)  [unwired: 5 in, 1 out]
                    n109 = call <vilib>:"Single Axis Load Velocity Override.vi"("error in (no error)"=w369, "Override Velosity Value"=w359, "Axis Select"=Axis_Select."Axis 2", "GECO Motion in"=w370) -> ("error out"=w367:errorcluster, "GECO Motion out"=w368:refnum<class "GECO Motion.lvclass">)  [unwired: 5 in, 1 out]
                    n110 = call <vilib>:"Single Axis Load Velocity Override.vi"("error in (no error)"=w367, "Override Velosity Value"=w359, "Axis Select"=Axis_Select."Axis 3", "GECO Motion in"=w368) -> ("error out"=w365:errorcluster, "GECO Motion out"=w366:refnum<class "GECO Motion.lvclass">)  [unwired: 5 in, 1 out]
                    n111 = call <vilib>:"MultiAxes Sync Move Start.vi"("error in (no error)"=w365, "Start Axes Select"=w360, "GECO Motion in"=w366) -> ("error out"=w371:errorcluster, "GECO Motion out"=w372:refnum<class "GECO Motion.lvclass">)  [unwired: 7 in]
                  }
                }
              }
              frame 7 {
                n112 = Unbundle By Name(w374) -> ("三軸同退"=w373:bool)
                n113 = case shown="False" w373 {
                  tunnel: w379 -> [w383 w403]
                  tunnel: w378 -> [w384 w402]
                  tunnel: w377 -> [_ w396]
                  tunnel: [w381 w411] -> w376
                  tunnel: [w380 w410] -> w375
                  frame False {
                    w382 = T4[] [enum."Axis 1", enum."Axis 2", enum."Axis 3"] items=["Axis 1", "Axis 2", "Axis 3", "Axis 4"] ("Start Axes Select")
                    n114 = for {
                      tunnel: w384 -> [w393]
                      tunnel: w383 -> [w392]
                      tunnel: w382 -> [w391] mode=indexing
                      tunnel: [w386] -> w381
                      tunnel: [w387] -> w380
                      w394 = u16 0 items=["Decelerate", "Halt"] ("Motion Stop Type")
                      n115 = call <vilib>:"Single Axis Move Stop.vi"("error in (no error)"=w393, "Motion Stop Type"=w394, "Axis Select"=w391, "GECO Motion in"=w392) -> ("error out"=w389:errorcluster, "Axis Select out"=w388:T4, "GECO Motion out"=w390:refnum<class "GECO Motion.lvclass">)  [unwired: 5 in]
                      n116 = call <vilib>:"Single Axis Load Velocity Override.vi"("error in (no error)"=w389, "Override Velosity Value"=0, "Axis Select"=w388, "GECO Motion in"=w390) -> ("error out"=w387:errorcluster, "GECO Motion out"=w386:refnum<class "GECO Motion.lvclass">)  [unwired: 5 in, 1 out]
                    }
                  }
                  frame True {
                    w399 = T4[] [enum."Axis 1", enum."Axis 2", enum."Axis 3"] items=["Axis 1", "Axis 2", "Axis 3", "Axis 4"] ("Start Axes Select")
                    n117 = Multiply(x=w396, y=-1) -> (x*y=w397:i32)
                    n118 = call <vilib>:"Single Axis Load Velocity Override.vi"("error in (no error)"=w402, "Override Velosity Value"=w397, "Axis Select"=Axis_Select."Axis 1", "GECO Motion in"=w403) -> ("error out"=w408:errorcluster, "GECO Motion out"=w409:refnum<class "GECO Motion.lvclass">)  [unwired: 5 in, 1 out]
                    n119 = call <vilib>:"Single Axis Load Velocity Override.vi"("error in (no error)"=w408, "Override Velosity Value"=w397, "Axis Select"=Axis_Select."Axis 2", "GECO Motion in"=w409) -> ("error out"=w406:errorcluster, "GECO Motion out"=w407:refnum<class "GECO Motion.lvclass">)  [unwired: 5 in, 1 out]
                    n120 = call <vilib>:"Single Axis Load Velocity Override.vi"("error in (no error)"=w406, "Override Velosity Value"=w397, "Axis Select"=Axis_Select."Axis 3", "GECO Motion in"=w407) -> ("error out"=w404:errorcluster, "GECO Motion out"=w405:refnum<class "GECO Motion.lvclass">)  [unwired: 5 in, 1 out]
                    n121 = call <vilib>:"MultiAxes Sync Move Start.vi"("error in (no error)"=w404, "Start Axes Select"=w399, "GECO Motion in"=w405) -> ("error out"=w410:errorcluster, "GECO Motion out"=w411:refnum<class "GECO Motion.lvclass">)  [unwired: 7 in]
                  }
                }
              }
            }
            n122 = Bundle By Name(cluster=w126, "GECO Motion out"=w127) -> (w132:T3)
          }
          frame "ZABMove" {
            w413 = T4[] [enum."Axis 1", enum."Axis 2", enum."Axis 3"] items=["Axis 1", "Axis 2", "Axis 3", "Axis 4"] ("Start Axes Select")
            n123 = Unbundle By Name(w424) -> ("PIDSetting.Move Setting"=w425:T9, "GECO Motion out"=w414:refnum<class "GECO Motion.lvclass">)
            n124 = call <vilib>:"MultiAxes Sync Move Start.vi"("error in (no error)"=w415, "Start Axes Select"=w413, "GECO Motion in"=w414) -> ("error out"=w416:errorcluster, "GECO Motion out"=w417:refnum<class "GECO Motion.lvclass">)  [unwired: 7 in]
            n125 = case shown="1" w425 {
              selector: w425 -> [_ w440 w547 _ _]
              tunnel: w424 -> [_ w462 w544 w550 w553]
              tunnel: w416 -> [w430 w471 w546 w549 w552]
              tunnel: [w429 w437 w498 w549 w552] -> w423
              tunnel: [w428 w441 w499 w548 w551] -> w421
              tunnel: [_ _ w485 _ _] -> w420
              tunnel: [_ _ w484 _ _] -> w419
              tunnel: [_ _ w483 _ _] -> w418
              tunnel: w417 -> [w426 _ w545 _ _]
              tunnel: [_ _ w486 _ _] -> w412
              frame Default {
                w427 = T4[] [enum."Axis 1", enum."Axis 2", enum."Axis 3", enum."Axis 4"] items=["Axis 1", "Axis 2", "Axis 3", "Axis 4"]
                n126 = for {
                  tunnel: w430 -> [w433]
                  tunnel: [w431] -> w429
                  tunnel: [w432] -> w428
                  tunnel: w427 -> [w435] mode=indexing
                  tunnel: w426 -> [w436]
                  w434 = u16 0 items=["Decelerate", "Halt"] ("Motion Stop Type")
                  n127 = call <vilib>:"Single Axis Move Stop.vi"("error in (no error)"=w433, "Motion Stop Type"=w434, "Axis Select"=w435, "GECO Motion in"=w436) -> ("error out"=w431:errorcluster, "GECO Motion out"=w432:refnum<class "GECO Motion.lvclass">)  [unwired: 5 in, 1 out]
                }
              }
              frame 0 {
                w450 = T4[] [enum."Axis 1", enum."Axis 2", enum."Axis 3"] items=["Axis 1", "Axis 2", "Axis 3", "Axis 4"] ("Start Axes Select")
                # "輸入Z、A、B"
                n128 = Unbundle By Name(w462) -> ("PIDSetting.Z"=w468:i32, "PIDSetting.A"=w467:i32, "PIDSetting.B"=w466:i32, "PIDSetting.Axis Length"=w476:dbl, "PIDSetting.Axis Pulse"=w472:dbl, "GECO Motion out"=w470:refnum<class "GECO Motion.lvclass">)
                n129 = Unbundle By Name(w462) -> ("ServoSetting.Singel Axis Move Paramters.Velocity (10000)"=w445:i32)
                n130 = call "綜合圓軌跡子VI.vi"("Ring"=w440, "移動z"=w468, "al"=w467, "be"=w466) -> ("Z"=w442:dbl, "A"=w443:dbl, "B"=w444:dbl)  [unwired: 2 in]
                n131 = call "推導公式.vi"("be"=w444, "al"=w443, "移動z"=w442) -> ("L3"=w477:dbl, "L2"=w478:dbl, "L1"=w479:dbl)
                n132 = Subtract(x=w479, y=w476) -> (x-y=w475:dbl)
                n133 = Subtract(x=w478, y=w476) -> (x-y=w474:dbl)
                n134 = Subtract(x=w477, y=w476) -> (x-y=w473:dbl)
                n135 = Multiply(x=w475, y=w472) -> (x*y=w438:dbl)
                n136 = Multiply(x=w474, y=w472) -> (x*y=w447:dbl)
                n137 = Multiply(x=w473, y=w472) -> (x*y=w439:dbl)
                n138 = call <vilib>:"Single Axis Load Velocity Override.vi"("error in (no error)"=w471, "Override Velosity Value"=w445, "Axis Select"=Axis_Select."Axis 1" ("Single Axis Select"), "GECO Motion in"=w470) -> ("error out"=w464:errorcluster, "Axis Select out"=w463:T4, "GECO Motion out"=w465:refnum<class "GECO Motion.lvclass">)  [unwired: 5 in]
                n139 = call <vilib>:"Single Axis Load Position Override.vi"("error in (no error)"=w464, "Override Target Position Value"=w439, "Axis Select"=w463, "GECO Motion in"=w465) -> ("error out"=w460:errorcluster, "GECO Motion out"=w461:refnum<class "GECO Motion.lvclass">)  [unwired: 5 in, 1 out]
                n140 = call <vilib>:"Single Axis Load Velocity Override.vi"("error in (no error)"=w460, "Override Velosity Value"=w445, "Axis Select"=Axis_Select."Axis 2" ("Single Axis Select"), "GECO Motion in"=w461) -> ("error out"=w457:errorcluster, "Axis Select out"=w456:T4, "GECO Motion out"=w458:refnum<class "GECO Motion.lvclass">)  [unwired: 5 in]
                n141 = call <vilib>:"Single Axis Load Position Override.vi"("error in (no error)"=w457, "Override Target Position Value"=w447, "Axis Select"=w456, "GECO Motion in"=w458) -> ("error out"=w451:errorcluster, "GECO Motion out"=w452:refnum<class "GECO Motion.lvclass">)  [unwired: 5 in, 1 out]
                n142 = call <vilib>:"Single Axis Load Velocity Override.vi"("error in (no error)"=w451, "Override Velosity Value"=w445, "Axis Select"=Axis_Select."Axis 3" ("Single Axis Select"), "GECO Motion in"=w452) -> ("error out"=w454:errorcluster, "Axis Select out"=w453:T4, "GECO Motion out"=w455:refnum<class "GECO Motion.lvclass">)  [unwired: 5 in]
                n143 = call <vilib>:"Single Axis Load Position Override.vi"("error in (no error)"=w454, "Override Target Position Value"=w438, "Axis Select"=w453, "GECO Motion in"=w455) -> ("error out"=w448:errorcluster, "GECO Motion out"=w449:refnum<class "GECO Motion.lvclass">)  [unwired: 5 in, 1 out]
                n144 = call <vilib>:"MultiAxes Sync Move Start.vi"("error in (no error)"=w448, "Start Axes Select"=w450, "GECO Motion in"=w449) -> ("error out"=w437:errorcluster, "GECO Motion out"=w441:refnum<class "GECO Motion.lvclass">)  [unwired: 7 in]
              }
              frame 1 {
                w543 = cluster{"output high":dbl, "output low":dbl} {"output high"=200000.0, "output low"=-500000.0} ("PID Def Output range")
                w511 = Axis_Select."Axis 3" ("Single Axis Select")
                w512 = Axis_Select."Axis 2" ("Single Axis Select")
                w510 = Axis_Select."Axis 1" ("Single Axis Select")
                # "PID取樣時間"
                # "Stm32 Delay Time"
                # "圓軌跡"
                n145 = Unbundle By Name(w544) -> ("PIDSetting.Axis Length"=w519:dbl, "PIDSetting.Axis Pulse"=w533:dbl)
                n146 = feedback #1() -> (w490:i32)
                n147 = Increment(x=w490) -> (x+1=w491:i32)
                n148 = feedback-in #1(w491) -> ()
                n149 = call <vilib>:"Read Encoder Position.vi"("error in (no error)"=w546, "Axis Select"=w510, "GECO Motion in"=w545) -> ("error out"=w517:errorcluster, "GECO Motion out"=w518:refnum<class "GECO Motion.lvclass">, "Encoder Position"=w497:i32, "Logical Position"=w509:i32)  [unwired: 4 in, 1 out]
                n150 = call <vilib>:"Read Encoder Position.vi"("error in (no error)"=w517, "Axis Select"=w512, "GECO Motion in"=w518) -> ("error out"=w515:errorcluster, "GECO Motion out"=w516:refnum<class "GECO Motion.lvclass">, "Encoder Position"=w496:i32, "Logical Position"=w508:i32)  [unwired: 4 in, 1 out]
                n151 = Bundle("Encoder Position"=w497, "Logical Position"=w509) -> (w485:T1)  [unwired: 1 in]
                n152 = call <vilib>:"Read Encoder Position.vi"("error in (no error)"=w515, "Axis Select"=w511, "GECO Motion in"=w516) -> ("error out"=w513:errorcluster, "GECO Motion out"=w514:refnum<class "GECO Motion.lvclass">, "Encoder Position"=w495:i32, "Logical Position"=w507:i32)  [unwired: 4 in, 1 out]
                n153 = call "綜合圓軌跡子VI.vi"("Ring"=w547, "I時間"=w490) -> ("Z"=w540:dbl, "A"=w489:dbl, "B"=w488:dbl)  [unwired: 4 in]
                n154 = property on="Axis 1" class="Clust (strict)"("Value"=w485) -> ()  [unwired: 2 in, 2 out]
                n155 = call "推導公式.vi"("be"=w488, "al"=w489, "移動z"=w540) -> ("L3"=w534:dbl, "L2"=w535:dbl, "L1"=w536:dbl)
                n156 = shared-variable "My Computer\\PC_Variables.lvlib\\PID gains"() -> (w482:T23)  [unwired: 1 in, 1 out]
                n157 = shared-variable "My Computer\\PC_Variables.lvlib\\PID gains 2"() -> (w481:T23)  [unwired: 1 in, 1 out]
                n158 = shared-variable "My Computer\\PC_Variables.lvlib\\PID gains 3"() -> (w480:T23)  [unwired: 1 in, 1 out]
                n159 = Bundle("Encoder Position"=w496, "Logical Position"=w508) -> (w484:T1)  [unwired: 1 in]
                n160 = Subtract(x=w536, y=w519) -> (x-y=w539:dbl)
                n161 = Subtract(x=w535, y=w519) -> (x-y=w538:dbl)
                n162 = Subtract(x=w534, y=w519) -> (x-y=w537:dbl)
                n163 = property on="Axis 2" class="Clust (strict)"("Value"=w484) -> ()  [unwired: 2 in, 2 out]
                n164 = feedback #2() -> (w494:i32)
                n165 = feedback-in #2(w497) -> ()
                n166 = feedback #3() -> (w493:i32)
                n167 = feedback-in #3(w496) -> ()
                n168 = feedback #4() -> (w492:i32)
                n169 = feedback-in #4(w495) -> ()
                n170 = Multiply ("L1 pulse")(x=w539, y=w533) -> (x*y=w505:dbl)
                n171 = Multiply ("L2 pulse")(x=w538, y=w533) -> (x*y=w504:dbl)
                n172 = Multiply ("L3 pulse")(x=w537, y=w533) -> (x*y=w503:dbl)
                n173 = Divide(x=25.0, y=1000.0) -> (x/y=w532:dbl)
                n174 = Bundle("Encoder Position"=w495, "Logical Position"=w507) -> (w483:T1)  [unwired: 1 in]
                n175 = property on="Axis 3" class="Clust (strict)"("Value"=w483) -> ()  [unwired: 2 in, 2 out]
                n176 = call-poly <vilib>:"PID.vi"("output range"=w543, "dt (s)"=w532, "PID gains"=w482, "process variable"=w494, "setpoint"=w503) -> ("output"=w502:dbl)  [unwired: 5 in, 1 out]
                n177 = call-poly <vilib>:"PID.vi"("output range"=w543, "dt (s)"=w532, "PID gains"=w481, "process variable"=w493, "setpoint"=w504) -> ("output"=w501:dbl)  [unwired: 5 in, 1 out]
                n178 = call-poly <vilib>:"PID.vi"("output range"=w543, "dt (s)"=w532, "PID gains"=w480, "process variable"=w492, "setpoint"=w505) -> ("output"=w500:dbl)  [unwired: 5 in, 1 out]
                n179 = call <vilib>:"Single Axis Load Velocity Override.vi"("error in (no error)"=w513, "Override Velosity Value"=w502, "Axis Select"=w510, "GECO Motion in"=w514) -> ("error out"=w530:errorcluster, "Axis Select out"=w522:T4, "GECO Motion out"=w531:refnum<class "GECO Motion.lvclass">)  [unwired: 5 in]
                n180 = call <vilib>:"Single Axis Load Position Override.vi"("error in (no error)"=w530, "Axis Select"=w522, "GECO Motion in"=w531) -> ("error out"=w528:errorcluster, "GECO Motion out"=w529:refnum<class "GECO Motion.lvclass">)  [unwired: 6 in, 1 out]
                n181 = shared-variable "My Computer\\PC_Variables.lvlib\\Axis 1 Position"(w485) -> ()  [unwired: 1 in, 1 out]
                n182 = call <vilib>:"Single Axis Load Velocity Override.vi"("error in (no error)"=w528, "Override Velosity Value"=w501, "Axis Select"=w512, "GECO Motion in"=w529) -> ("error out"=w506:errorcluster, "Axis Select out"=w521:T4, "GECO Motion out"=w527:refnum<class "GECO Motion.lvclass">)  [unwired: 5 in]
                n183 = call <vilib>:"Single Axis Load Position Override.vi"("error in (no error)"=w506, "Axis Select"=w521, "GECO Motion in"=w527) -> ("error out"=w525:errorcluster, "GECO Motion out"=w526:refnum<class "GECO Motion.lvclass">)  [unwired: 6 in, 1 out]
                n184 = call <vilib>:"Single Axis Load Velocity Override.vi"("error in (no error)"=w525, "Override Velosity Value"=w500, "Axis Select"=w511, "GECO Motion in"=w526) -> ("error out"=w523:errorcluster, "Axis Select out"=w520:T4, "GECO Motion out"=w524:refnum<class "GECO Motion.lvclass">)  [unwired: 5 in]
                n185 = shared-variable "My Computer\\PC_Variables.lvlib\\Axis 2 Position"(w484) -> ()  [unwired: 1 in, 1 out]
                n186 = call <vilib>:"Single Axis Load Position Override.vi"("error in (no error)"=w523, "Axis Select"=w520, "GECO Motion in"=w524) -> ("error out"=w498:errorcluster, "GECO Motion out"=w499:refnum<class "GECO Motion.lvclass">)  [unwired: 6 in, 1 out]
                n187 = shared-variable "My Computer\\PC_Variables.lvlib\\Axis 3 Position"(w483) -> ()  [unwired: 1 in, 1 out]
                n188 = Bundle By Name(cluster=cluster{"A":dbl, "B":dbl} {"A"=0.0, "B"=0.0} ("理想角度"), "A"=w489, "B"=w488) -> (w486:cluster{"A":dbl, "B":dbl})
              }
              frame 2 {
                # "Á³±Û­y¸ñ"
                n189 = Unbundle By Name(w550) -> ("GECO Motion out"=w548:refnum<class "GECO Motion.lvclass">)
              }
              frame 3 {
                # "Z上下"
                n190 = Unbundle By Name(w553) -> ("GECO Motion out"=w551:refnum<class "GECO Motion.lvclass">)
              }
            }
            n191 = Bundle By Name(cluster=w424, "GECO Motion out"=w421, "Axis 1 Position"=w420, "Axis 2 Position"=w419, "Axis 3 Position"=w418, "理想角度"=w412) -> (w422:T3)
          }
          frame "AlarmReset" {
            w560 = T4[] [enum."Axis 1", enum."Axis 2", enum."Axis 3", enum."Axis 4"] items=["Axis 1", "Axis 2", "Axis 3", "Axis 4"]
            n192 = Unbundle By Name(w559) -> ("GECO Motion out"=w557:refnum<class "GECO Motion.lvclass">)
            n193 = for {
              tunnel: [w569] -> w555
              tunnel: [w568] -> w554
              tunnel: w560 -> [w563] mode=indexing
              tunnel: w558 -> [w565]
              tunnel: w557 -> [w564]
              w561 = u16 0 items=["Decelerate", "Halt"] ("Motion Stop Type")
              n194 = call <vilib>:"Single Axis Move Stop.vi"("error in (no error)"=w565, "Motion Stop Type"=w561, "Axis Select"=w563, "GECO Motion in"=w564) -> ("error out"=w566:errorcluster, "Axis Select out"=w562:T4, "GECO Motion out"=w567:refnum<class "GECO Motion.lvclass">)  [unwired: 5 in]
              n195 = call <vilib>:"Alarm Reset.vi"("error in (no error)"=w566, "Axis Select"=w562, "GECO Motion in"=w567) -> ("error out"=w568:errorcluster, "GECO Motion out"=w569:refnum<class "GECO Motion.lvclass">)  [unwired: 6 in, 1 out]
            }
            n196 = Bundle By Name(cluster=w559, "GECO Motion out"=w555) -> (w556:T3)
          }
          frame "EncoderReset" {
            w576 = T4[] [enum."Axis 1", enum."Axis 2", enum."Axis 3", enum."Axis 4"] items=["Axis 1", "Axis 2", "Axis 3", "Axis 4"]
            n197 = Unbundle By Name(w575) -> ("GECO Motion out"=w573:refnum<class "GECO Motion.lvclass">)
            n198 = for {
              tunnel: [w585] -> w571
              tunnel: [w584] -> w570
              tunnel: w576 -> [w583] mode=indexing
              tunnel: w574 -> [w580]
              tunnel: w573 -> [w579]
              w577 = u16 0 items=["Decelerate", "Halt"] ("Motion Stop Type")
              n199 = call <vilib>:"Single Axis Move Stop.vi"("error in (no error)"=w580, "Motion Stop Type"=w577, "Axis Select"=w583, "GECO Motion in"=w579) -> ("error out"=w581:errorcluster, "Axis Select out"=w578:T4, "GECO Motion out"=w582:refnum<class "GECO Motion.lvclass">)  [unwired: 5 in]
              n200 = call <vilib>:"Reset Encoder Position.vi"("error in (no error)"=w581, "Axis Select"=w578, "GECO Motion in"=w582) -> ("error out"=w584:errorcluster, "GECO Motion out"=w585:refnum<class "GECO Motion.lvclass">)  [unwired: 6 in, 1 out]
            }
            n201 = Bundle By Name(cluster=w575, "GECO Motion out"=w571) -> (w572:T3)
          }
          frame "LinkBoard" {
            n202 = Unbundle By Name(w606) -> ("resource name"=w596:tag, "TCP slave port"=w604:u16, "ServoSetting.Motion Controller Slot"=w597:T7)
            n203 = Format Date/Time String(time format string (%c)="%Y %m %d %H %M ") -> (date/time string=w593:string)  [unwired: 2 in]
            n204 = Concatenate Strings(w593, "Ideal Angle.txt" ("element")) -> (w592:string)
            n205 = Build Path(base path=path "u:/data", name or relative path=w592) -> (appended path=w594:path)
            n206 = Open/Create/Replace File(file path (use dialog)=w594, error in=w588, operation (0:open)=T19."replace or create") -> (refnum out=w586:refnum<file>, error out=w589:errorcluster)  [unwired: 3 in, 1 out]
            n207 = call-poly <vilib>:"Create Modbus Instance.vi"("error in"=w589, "port (502)"=w604) -> ("error out"=w603:errorcluster, "TCP slave instance"=w598:refnum<class "Modbus Slave.lvclass">)  [unwired: 8 in]
            n208 = call-poly <vilib>:"InitializeRT.vi"("error in (no error)"=w603, "resource name"=w596) -> ("error out"=w602:errorcluster, "GECO_Driver out"=w599:refnum<class "GECO_Driver.lvclass">)  [unwired: 8 in]
            n209 = call <vilib>:"Initialize Motion Controller.vi"("error in (no error)"=w602, "Slot"=w597, "GECO_Driver in"=w599) -> ("error out"=w600:errorcluster, "Motion reference out"=w601:refnum<class "GECO Motion.lvclass">)  [unwired: 7 in]
            n210 = Bundle By Name(cluster=w606, "Modbus COM"=w598, "GECO_Driver out"=w599, "GECO Motion out"=w601, "Save Path"=w586) -> (w605:T3)
          }
          frame "PanelUpdate" {
            n211 = Unbundle By Name(w629) -> ("GECO Motion out"=w628:refnum<class "GECO Motion.lvclass">)
            n212 = call <vilib>:"Read Encoder Position.vi"("error in (no error)"=w631, "Axis Select"=Axis_Select."Axis 1", "GECO Motion in"=w628) -> ("error out"=w624:errorcluster, "GECO Motion out"=w625:refnum<class "GECO Motion.lvclass">, "Encoder Position"=w617:i32, "Logical Position"=w618:i32)  [unwired: 4 in, 1 out]
            n213 = Bundle(cluster=T20 {"Logical Position"=0, "Encoder Position"=0} ("input cluster"), "Logical Position"=w618, "Encoder Position"=w617) -> (w609:T20)
            "Axis 1" <- w609
            n214 = shared-variable "My Computer\\PC_Variables.lvlib\\Axis 1 Position"(w609) -> ()  [unwired: 1 in, 1 out]
            n215 = call <vilib>:"Read Encoder Position.vi"("error in (no error)"=w624, "Axis Select"=Axis_Select."Axis 2", "GECO Motion in"=w625) -> ("error out"=w622:errorcluster, "GECO Motion out"=w623:refnum<class "GECO Motion.lvclass">, "Encoder Position"=w610:i32, "Logical Position"=w611:i32)  [unwired: 4 in, 1 out]
            n216 = Bundle(cluster=T20 {"Logical Position"=0, "Encoder Position"=0} ("input cluster"), "Logical Position"=w611, "Encoder Position"=w610) -> (w608:T20)
            "Axis 2" <- w608
            n217 = shared-variable "My Computer\\PC_Variables.lvlib\\Axis 2 Position"(w608) -> ()  [unwired: 1 in, 1 out]
            n218 = call <vilib>:"Read Encoder Position.vi"("error in (no error)"=w622, "Axis Select"=Axis_Select."Axis 3", "GECO Motion in"=w623) -> ("error out"=w630:errorcluster, "GECO Motion out"=w626:refnum<class "GECO Motion.lvclass">, "Encoder Position"=w612:i32, "Logical Position"=w613:i32)  [unwired: 4 in, 1 out]
            n219 = Bundle(cluster=T20 {"Logical Position"=0, "Encoder Position"=0} ("input cluster"), "Logical Position"=w613, "Encoder Position"=w612) -> (w607:T20)
            "Axis 3" <- w607
            n220 = shared-variable "My Computer\\PC_Variables.lvlib\\Axis 3 Position"(w607) -> ()  [unwired: 1 in, 1 out]
            n221 = Bundle By Name(cluster=w629, "GECO Motion out"=w626, "Axis 1 Position"=w609, "Axis 2 Position"=w608, "Axis 3 Position"=w607) -> (w627:T3)
          }
          frame "CloseBoard" {
            w635 = T4[] [enum."Axis 1", enum."Axis 2", enum."Axis 3", enum."Axis 4"] items=["Axis 1", "Axis 2", "Axis 3", "Axis 4"]
            n222 = RT FIFO Delete(0:w632, 3:w633) -> (11:w634:errorcluster)  [unwired: 1 in]
            n223 = Unbundle By Name(w640) -> ("GECO_Driver out"=w637:refnum<class "GECO_Driver.lvclass">, "GECO Motion out"=w636:refnum<class "GECO Motion.lvclass">)
            n224 = for {
              tunnel: [w645] -> w638
              tunnel: w636 -> [w644]
              tunnel: w634 -> [w643]
              tunnel: w635 -> [w641] mode=indexing
              n225 = call <vilib>:"Servo On.vi"("error in (no error)"=w643, "Servo On"=FALSE, "Axis Select"=w641, "GECO Motion in"=w644) -> ("error out"=w648:errorcluster, "Axis Select out"=w647:T4, "GECO Motion out"=w646:refnum<class "GECO Motion.lvclass">)  [unwired: 5 in]
              n226 = call <vilib>:"Single Axis Move Stop.vi"("error in (no error)"=w648, "Axis Select"=w647, "GECO Motion in"=w646) -> ("error out"=w645:errorcluster)  [unwired: 6 in, 2 out]
            }
            n227 = call <vilib>:"Close.vi"("error in (no error)"=w638, "GECO_Driver in"=w637) -> ("error out"=w639:errorcluster)  [unwired: 9 in]
          }
        }
        "error out" <- w41
        n228 = shared-variable "NI-sbRIO9606-01F1BAB2\\RT_Variables.lvlib\\error out"(w41) -> ()  [unwired: 1 in, 1 out]
        n229 = Unbundle By Name(w41) -> ("status"=w42:bool)
      }
      frame Error {
      }
    }
    n230 = Tick Count (ms)() -> (millisecond timer value=w33:u32)
    n231 = Unbundle By Name(w31) -> ("理想角度"=w30:cluster{"A":dbl, "B":dbl})
    n232 = Subtract(x=w33, y=w32) -> (x-y=w29:u32)
    "Program Period" <- w29
    n233 = shared-variable "NI-sbRIO9606-01F1BAB2\\RT_Variables.lvlib\\Program Period"(w29) -> ()  [unwired: 1 in, 1 out]
    n234 = node-c288() -> ()  [unwired: 1 in, 1 out]
  }
  n235 = node-c288(w7) -> ()  [unwired: 1 out]
  n236 = Unbundle By Name(w11) -> ("Save Path"=w10:refnum<file>)
  n237 = for {
    tunnel: [w661] -> w9 mode=indexing
    tunnel: w13 -> [w660] mode=indexing
    tunnel: w12 -> [w657] mode=indexing
    n238 = Unbundle(w660) -> ("A"=w659:dbl, "B"=w658:dbl)
    n239 = Format Into String(w659) -> (resulting string=w654:string)  [unwired: 3 in, 1 out]
    n240 = Format Into String(w658) -> (resulting string=w652:string)  [unwired: 3 in, 1 out]
    n241 = Format Into String(w657) -> (resulting string=w656:string)  [unwired: 3 in, 1 out]
    n242 = Insert Into Array(array=string[] ["Program Period(ms)："], new element #1=w656, new element #2="A：", new element #3=w654, new element #4="B：", new element #5=w652) -> (w661:string[])  [unwired: 1 in]
  }
  n243 = for {
    tunnel: w9 -> [w665] mode=indexing
    shift-right: [w663] -> _
    shift-left: w10 -> [w667]
    shift-right: [w664] -> _
    shift-left: _ -> [w666]
    n244 = Array To Spreadsheet String(delimiter (Tab)="\t", array=w665, 3:"%f" ("format string")) -> (spreadsheet string=w668:string)
    n245 = Write to Text File(file (use dialog)=w667, text=w668, error in=w666) -> (refnum out=w663:refnum<file>, error out=w664:errorcluster)  [unwired: 1 in, 1 out]
  }
